vi "Set VISA DBL output.vi"(7 "VISA resource name":refnum<visa-resource-name>, 8 "error in (no error)":errorcluster, 9 "Output value":dbl, 10 "Mag Lab Parameters in":refnum<class "Mag Lab Parameters.lvclass">, 11 "Visa instrument in":refnum<class "Visa instrument.lvclass">) -> (0 "error out":errorcluster, 1 "Actula output value":dbl, 3 "Visa instrument out":refnum<class "Visa instrument.lvclass">, 5 "VISA resource name out":refnum<visa-resource-name>)   [LabVIEW 2015, in "Visa instrument.lvclass"]
uses:
  Visa instrument.lvclass
  Mag Lab Properties/Mag Lab Parameters.lvclass
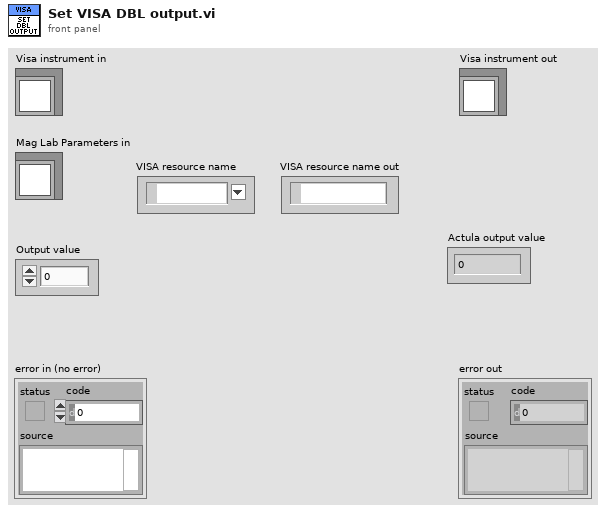
[diagram p1: front panel]
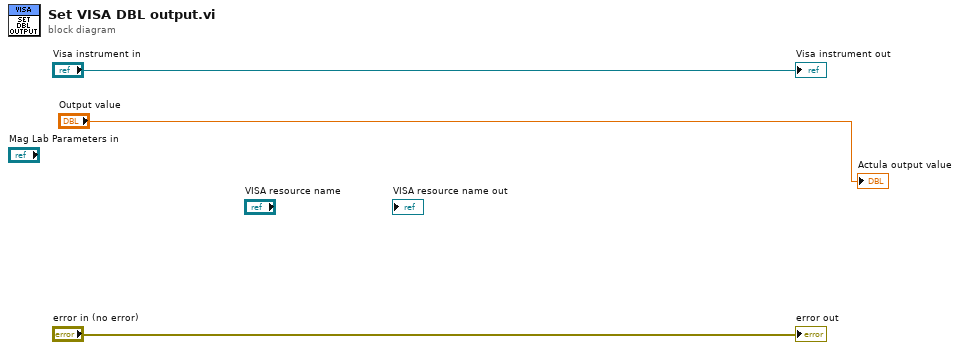
[diagram p0: block diagram]
diagram:
  "error out" <- "error in (no error)"
  "Visa instrument out" <- "Visa instrument in"
  "Actula output value" <- "Output value"
